vi "PDLM_GetQueuedErrorString.vi"(8 "error in (no error)":errorcluster, 10 "ErrCode":i32, 11 "USBIdx":i32) -> (0 "error out":errorcluster, 2 "ErrText":string, 3 "return type":i32)   [LabVIEW 2019]
uses:
  <userlib>/TaikoLaser/PDLM_DllPath_global.vi
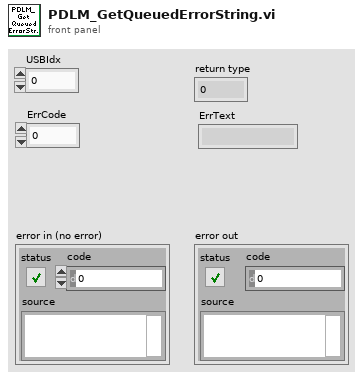
[diagram p1: front panel]
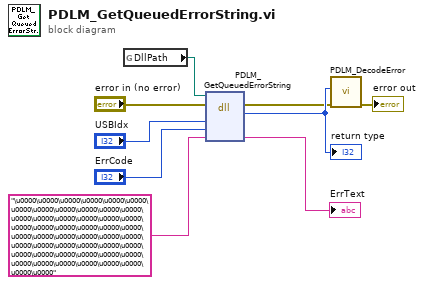
[diagram p0: block diagram]
diagram:
  n1 = global read "PDLM_DllPath_global.vi" "DllPath"() -> (w5:path)
  n2 = dll-call lib="M:/_dev/progs/LabVIEW/_lib/PQ/Taiko/pdlm_lib.dll" fn="PDLM_GetQueuedErrorString"(path in=w5, error in="error in (no error)", "USBIdx"="USBIdx", "ErrCode"="ErrCode", "ErrText"="\u0000\u0000\u0000\u0000\u0000\u0000\u0000\u0000\u0000\u0000\u0000\u0000\u0000\u0000\u0000\u0000\u0000\u0000\u0000\u0000\u0000\u0000\u0000\u0000\u0000\u0000\u0000\u0000\u0000\u0000\u0000\u0000\u0000\u0000\u0000\u0000\u0000\u0000\u0000\u0000\u0000\u0000\u0000\u0000\u0000\u0000\u0000\u0000\u0000\u0000") -> (error out=w7:errorcluster, "return type"=w8:i32, "ErrText"=→"ErrText":string)  [unwired: 3 in, 1 out]
  "return type" <- w8
  n3 = call <userlib>:"PDLM_DecodeError.vi"("error in (no error)"=w7, "code"=w8) -> ("error out"=→"error out":errorcluster)  [unwired: 7 in, 2 out]
